vi "Add Address to Command.vi"(1 "Address (0)":i32 min=0 max=16 step=1, 2 "Command":string) -> (0 "Command OUT":string)   [LabVIEW 2021, in "Environment Chamber.lvlib" / "Climatic Chamber.lvlib"]
uses:
  Climatic Chamber.lvlib
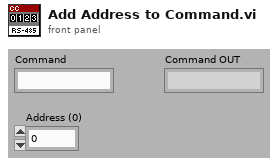
[diagram p1: front panel]
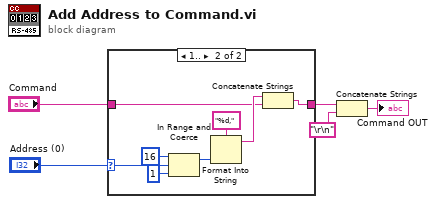
[diagram p0: block diagram]
diagram:
  n1 = case shown="1.." "Address (0)" {
    selector: "Address (0)" -> [_ w12]
    tunnel: [w6 w7] -> w4
    tunnel: "Command" -> [w6 w8]
    frame ..0 {
    }
    frame 1.. {
      n2 = In Range and Coerce(upper limit=16, x=w12, lower limit=1) -> (coerced(x)=w11:i32)  [unwired: 1 out]
      n3 = Format Into String(format string="%d,", w11) -> (resulting string=w9:string)  [unwired: 2 in, 1 out]
      n4 = Concatenate Strings(w9, w8) -> (w7:string)
    }
  }
  n5 = Concatenate Strings(w4, "\r\n") -> (→"Command OUT":string)
